vi "Disable Item.vi"(8 "error in (no error)":errorcluster, 10 "Item":refnum<class "Item.lvclass">, 11 "Listbox in":refnum<class "Listbox.lvclass">) -> (0 "error out":errorcluster, 3 "Listbox out":refnum<class "Listbox.lvclass">)   [LabVIEW 2016, in "斯坦道总磷总氮.lvlib" / "Listbox.lvclass"]
uses:
  Listbox.lvclass
  Interfaces/Item/Item.lvclass
  Listbox Item/Listbox Item.lvclass
  Listbox.lvclass/Listbox.ctl
  <vilib>/Utility/error.llb/Error Cluster From Error Code.vi
  <vilib>/ErrorRing/Error Ring.xnode
panel:
  # "NOTICE -- YOU MUST LEAVE THIS NOTICE IN PLACE.\n\nCopyright (c) 2017, LIANG LIU Shawn.Liu.cn@gmail.com\nAll rights reserved.\n\nRedistribution and use in source and binary forms, with or without modification, are permitted provided that the following conditions are met:\n-Redistributions of source code must retain the above copyright notice, this list of conditions and the following disclaimer.\n-Redistributions in binary form must reproduce the above copyright notice, this list of conditions and the following disclaimer in the documentation and/or other materials provided with the distribution.\n-Neither the name of the eLp nor the names of its contributors may be used to endorse or promote products derived from this software without specific prior written permission.\n\nTHIS SOFTWARE IS PROVIDED BY THE COPYRIGHT HOLDERS AND CONTRIBUTORS \"AS IS\" AND ANY EXPRESS OR IMPLIED WARRANTIES, INCLUDING, BUT NOT LIMITED TO, THE IMPLIED WARRANTIES OF MERCHANTABILITY AND FITNESS FOR A PARTICULAR PURPOSE ARE DISCLAIMED. IN NO EVENT SHALL THE COPYRIGHT HOLDER OR CONTRIBUTORS BE LIABLE FOR ANY DIRECT, INDIRECT, INCIDENTAL, SPECIAL, EXEMPLARY, OR CONSEQUENTIAL DAMAGES (INCLUDING, BUT NOT LIMITED TO, PROCUREMENT OF SUBSTITUTE GOODS OR SERVICES; LOSS OF USE, DATA, OR PROFITS; OR BUSINESS INTERRUPTION) HOWEVER CAUSED AND ON ANY THEORY OF LIABILITY, WHETHER IN CONTRACT, STRICT LIABILITY, OR TORT (INCLUDING NEGLIGENCE OR OTHERWISE) ARISING IN ANY WAY OUT OF THE USE OF THIS SOFTWARE, EVEN IF ADVISED OF THE POSSIBILITY OF SUCH DAMAGE."
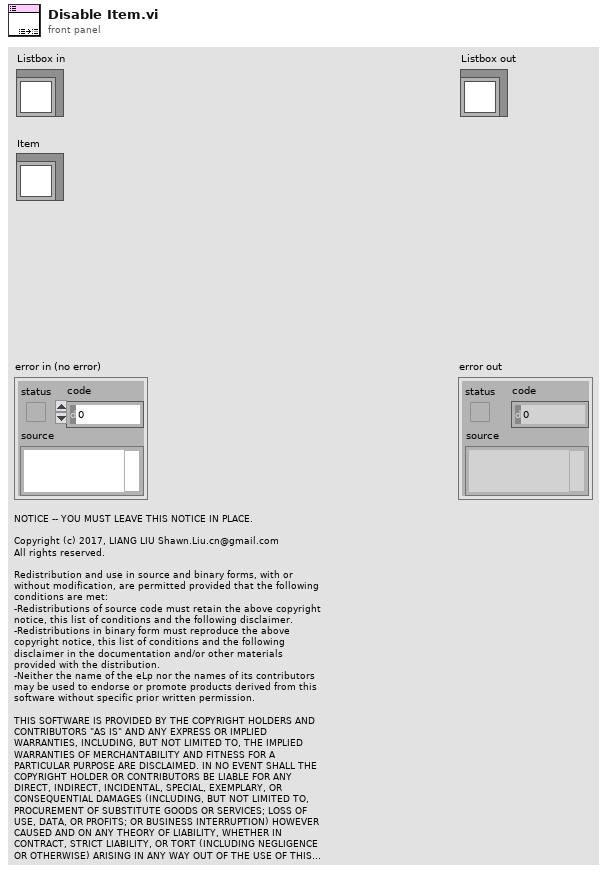
[diagram p1: front panel]
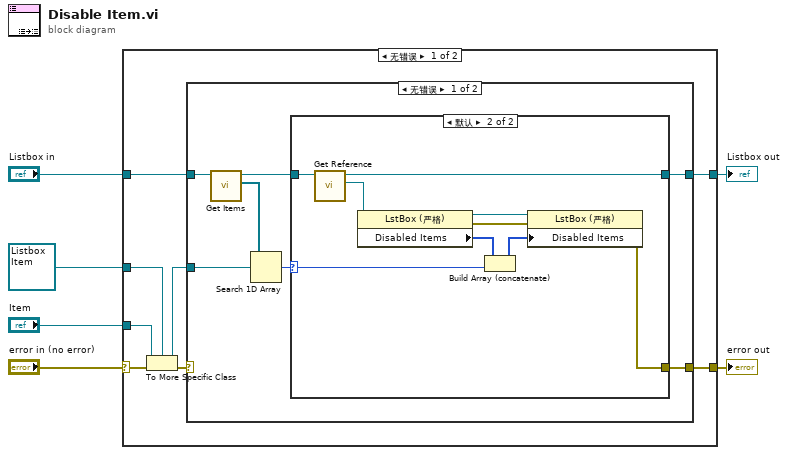
[diagram p0: block diagram]
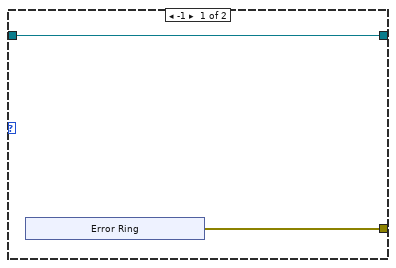
[diagram p2: hidden frame]
diagram:
  n1 = case shown="无错误" "error in (no error)" {
    selector: "error in (no error)" -> [w11 w40]
    tunnel: refnum<class "Listbox Item.lvclass"> refnum ("Listbox Item.lvclass") -> [w14 _]
    tunnel: "Listbox in" -> [w13 w39]
    tunnel: "Item" -> [w12 _]
    tunnel: [w10 w39] -> w2
    tunnel: [w9 w40] -> w1
    frame No Error {
      n2 = To More Specific Class(target class=w14, reference=w12, error in=w11) -> (specific class reference=w8:refnum<class "Listbox Item.lvclass">, error out=w7:errorcluster)
      n3 = case shown="无错误" w7 {
        selector: w7 -> [_ w38]
        tunnel: w13 -> [w21 w37]
        tunnel: [w20 w37] -> w10
        tunnel: [w19 w38] -> w9
        tunnel: w8 -> [w18 _]
        frame No Error {
          n4 = call "Get Items.vi"("Listbox in"=w21) -> ("Items"=w16:refnum<class "Listbox Item.lvclass">[], "Listbox out"=w17:refnum<class "Listbox.lvclass">)  [unwired: 9 in]
          n5 = Search 1D Array(1D array=w16, element=w18) -> (index of element=w15:i32)  [unwired: 1 in]
          n6 = case shown="默认" w15 {
            selector: w15 -> [_ w28]
            tunnel: [w23 w36] -> w20
            tunnel: [w22 w35] -> w19
            tunnel: w17 -> [w23 w34]
            frame -1 {
              n7 = xnode "Error Ring"() -> ("错误输出"=w22:errorcluster)
            }
            frame Default {
              n8 = call "Get Reference.vi"("Listbox in"=w34) -> ("Reference"=w32:refnum<vi>, "Listbox out"=w36:refnum<class "Listbox.lvclass">)  [unwired: 9 in]
              n9 = property class="LstBox (严格)"(reference=w32) -> (reference out=w33:refnum<vi>, error out=w31:errorcluster, "Disabled Items"=w30:i32[])  [unwired: 1 in]
              n10 = Build Array (concatenate)(w30, w28) -> (w29:i32[])
              n11 = property class="LstBox (严格)"(reference=w33, error in=w31, "Disabled Items"=w29) -> (error out=w35:errorcluster)  [unwired: 1 out]
            }
          }
        }
        frame Error {
        }
      }
    }
    frame Error {
    }
  }
  "error out" <- w1
  "Listbox out" <- w2
